vi "QCameraV1_0.vi"() -> (0 "stopped":bool)   [LabVIEW 2012]
uses:
  <vilib>/vision/Image Controls.llb/IMAQ Image.ctl
  SubVI/ProSCI Global.vi
  <userlib>/QI_Transition.llb/QCam Grab Abort.vi
  SubVI/ProSCI DebugGlobal.vi
  <userlib>/QCam Color Globals.vi
  <vilib>/vision/NI_Vision_Development_Module.lvlib
panel:
  out "Images Collected":u64
  in  "Blue Gain":u32=1 min=1 step=1
  in  "Red Gain":u32=1 min=1 step=1
  in  "Green Gain":u32=1 min=1 step=1
  in  "Blue Exposure":dbl=483.0
  in  "Red Exposure":dbl=235.0
  in  "Green Exposure":dbl=300.0
  out "Ratio BlueGreen FL":dbl
  out "Ratio RedGreen FL":dbl
  in  "Link Exposures (FL)":bool
  in  "ForwardDelay":dbl=0.04 min=0.04 max=1074000.0 step=0.001 format="%#.3f"
  in  "FLLampOffDelay":dbl=0.04 min=0.04 max=1074000.0 step=0.001 format="%#.3f"
  in  "FLLampOnDelay":dbl=0.04 min=0.04 max=1074000.0 step=0.001 format="%#.3f"
  in  "BFLampOffDelay":dbl=0.04 min=0.04 max=1074000.0 step=0.001 format="%#.3f"
  in  "BFLampOnDelay":dbl=0.04 min=0.04 max=1074000.0 step=0.001 format="%#.3f"
  in  "PreImagingDelay":dbl=0.04 min=0.04 max=1074000.0 step=0.001 format="%#.3f"
  out "FLExposureTime":dbl[](array[numeric]) caption="Set FL Exposure Time (ms)"
  out "CurrentExposureTime":dbl[](array[numeric]) caption="Current Camera\nExposure Time (ms)"
  in  "SetFLExposureTime":bool
  in  "SetBFExpsureTime":bool
  in  "FLExcite6":bool
  out "FLExciteLED6":bool
  in  "FLExcite5":bool
  out "FLExciteLED5":bool
  in  "FLExcite4":bool
  out "FLExciteLED4":bool
  in  "FLExcite3":bool
  out "FLExciteLED3":bool
  in  "FLExcite2":bool
  out "FLExciteLED2":bool
  in  "FLExcite1":bool
  out "FLExciteLED1":bool
  in  "FL Blue Exp":dbl=0.03999999910593033 min=0.03999999910593033 max=1074000.0 step=0.001 format="%#_3f"
  in  "FL Red Exp":dbl=0.04 min=0.04 max=1074000.0 step=0.001 format="%#.3f"
  in  "FL Exp":dbl=0.04 min=0.04 max=1074000.0 step=0.001 format="%#.3f"
  in  "Case Constant\n(See Context Help) 2":bool
  in  "Case Constant\n(See Context Help)":bool=TRUE
  out "Camera Trigger Mode":T1(ring)
  in  "qImage Type":enum32{"Color", "Grayscale"}(radio)
  out "Ratio BlueGreen":dbl
  out "Ratio RedGreen":dbl
  in  "Tab Control":T2(tab)
  in  "Show Real-Time Image":bool
  out "Real-Time Image":T3(plugin-control)
  in  "Last Or Last Last":enum32{"Last", "Last Last"}(radio)
  in  "Last Display Type":enum32{"Color", "Grayscale"}(radio)
  out "Last Image":T3(plugin-control)
  out "Stream":bool
  out "StatusgGrabImage":bool
  out "Last Last Color":T3
  out "Last Last Mono":T3
  out "Last ColorImage":T3
  out "Last MonoImage":T3
  out "ColorImage":T3
  out "MonoImage":T3
  in  "Snap":bool
  out "TypeChanged":bool
  out "FirstPass":bool
  out "qSerial No":string
  out "last image":errorcluster
  in  "Link Exposures (BF)":bool
  in  "User Blue Exp":dbl=0.03999999910593033 min=0.03999999910593033 max=1074000.0 step=0.001 format="%#_3f"
  in  "User Red Exp":dbl=0.04 min=0.04 max=1074000.0 step=0.001 format="%#.3f"
  in  "White Balance":bool
  in  "Auto Expose":bool
  in  "User Exp":dbl=0.04 min=0.04 max=1074000.0 step=0.001 format="%#.3f"
  in  "Stop Button":bool
  # "CAMERA DISPLAY"
  # "Fluorescence Excitation Filters"
  # "Choice"
  # "Active"
  # "Filter 1"
  # "Filter 2"
  # "Filter 3"
  # "Filter 4"
  # "Filter 5"
  # "Filter 6"
  # "Waiting Scheme (Addition to Exp Time)"
  # "Forward Delay"
  # "msec"
  # "Delay before\nImaging"
  # "msec"
  # "BF Lamp on Delay"
  # "msec"
  # "BF  Lamp off Delay"
  # "msec"
  # "FL  Lamp on Delay"
  # "msec"
  # "FL  Lamp off Delay"
  # "msec"
  # "msec"
  # "msec"
  # "BF Exposure"
  # "FL Exposure"
  # "BF Exposure (Red)"
  # "FL Exposure (Red)"
  # "msec"
  # "msec"
  # "msec"
  # "BF Exposure (Blue)"
  # "FL Exposure (Blue)"
  # "msec"
  # "Display"
  # "Image"
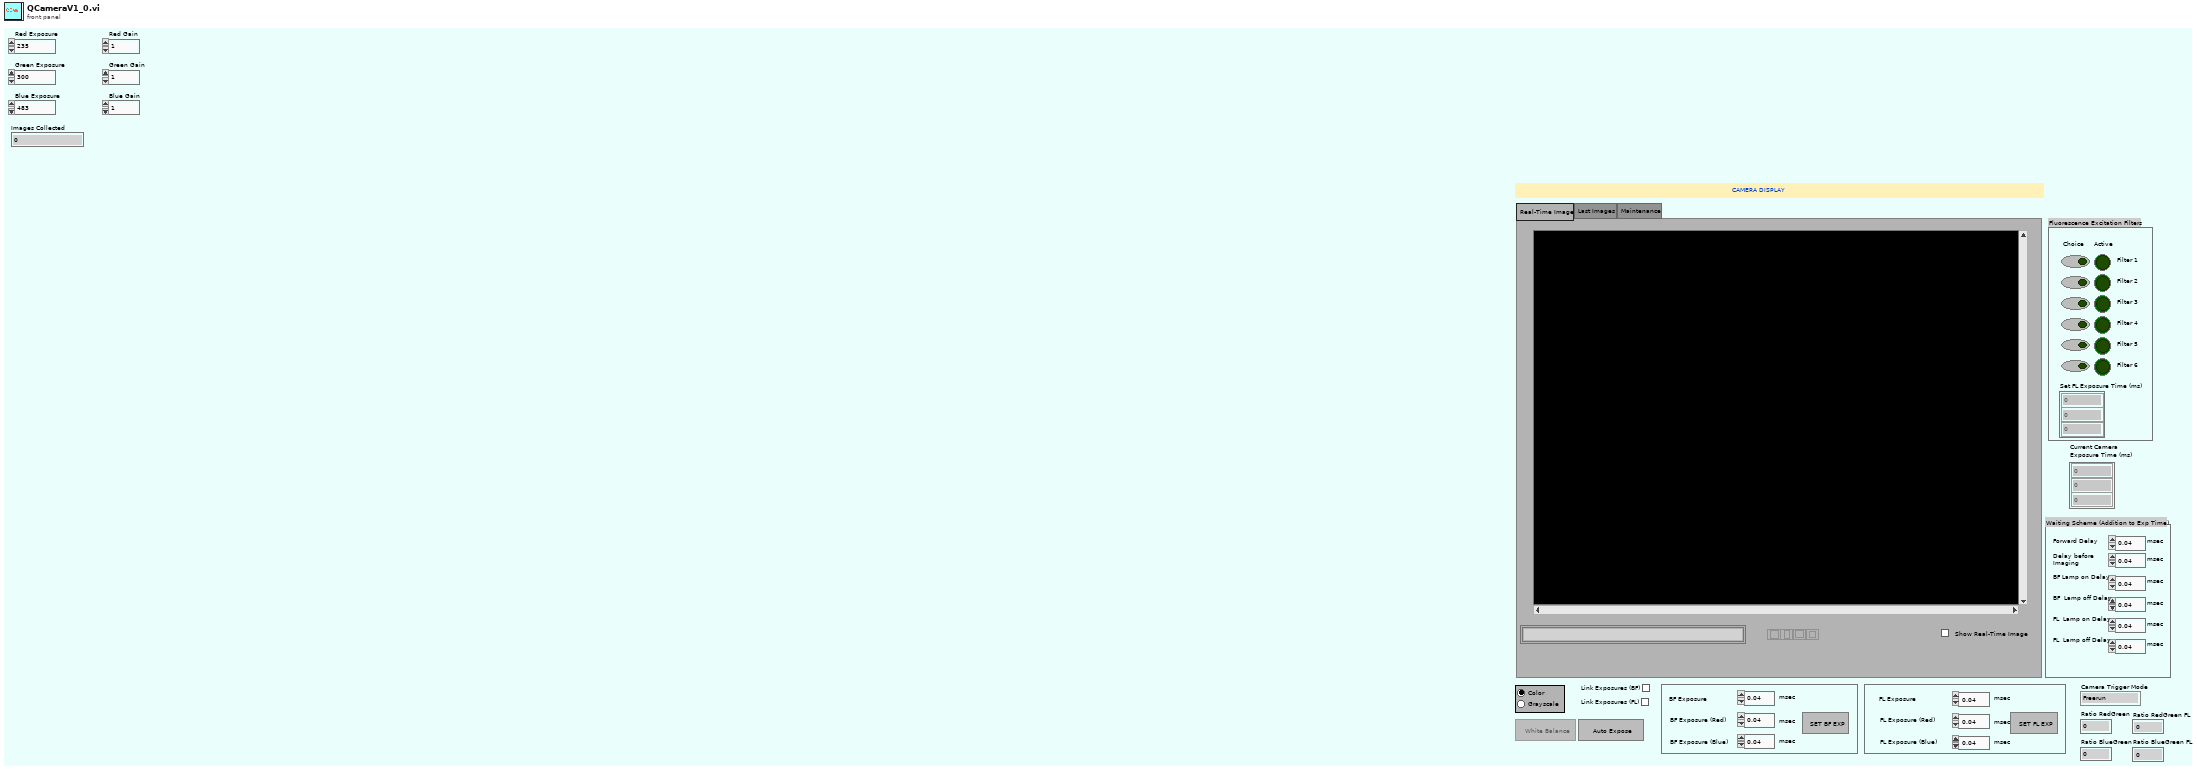
[diagram p1: front panel]
types:
  T1 = enum32{"Freerun", "Edge hi", "Edge low", "Pulse hi", "Pulse low", "Software"}
  T2 = enum32{"Real-Time Image", "Last Images", "Maintenance"}
  T3 = typedef "IMAQ Image.ctl" = refnum<image>
  T4 = typedef "LVRectTypeDef.ctl" = cluster{"Left":i16, "Top":i16, "Right":i16, "Bottom":i16}
  T5 = typedef "Image Type" = u32
  T6 = cluster{"Global Rectangle":i32[], "Contours":cluster{"Contour Type":u32, "ROI Type":u32, "Points":i32[]}[]}
  T7 = cluster{"Green Gain":u32, "Red Gain":u32, "Blue Gain":u32}
  T8 = cluster{"Green Exposure":dbl, "Red Exposure":dbl, "Blue Exposure":dbl}
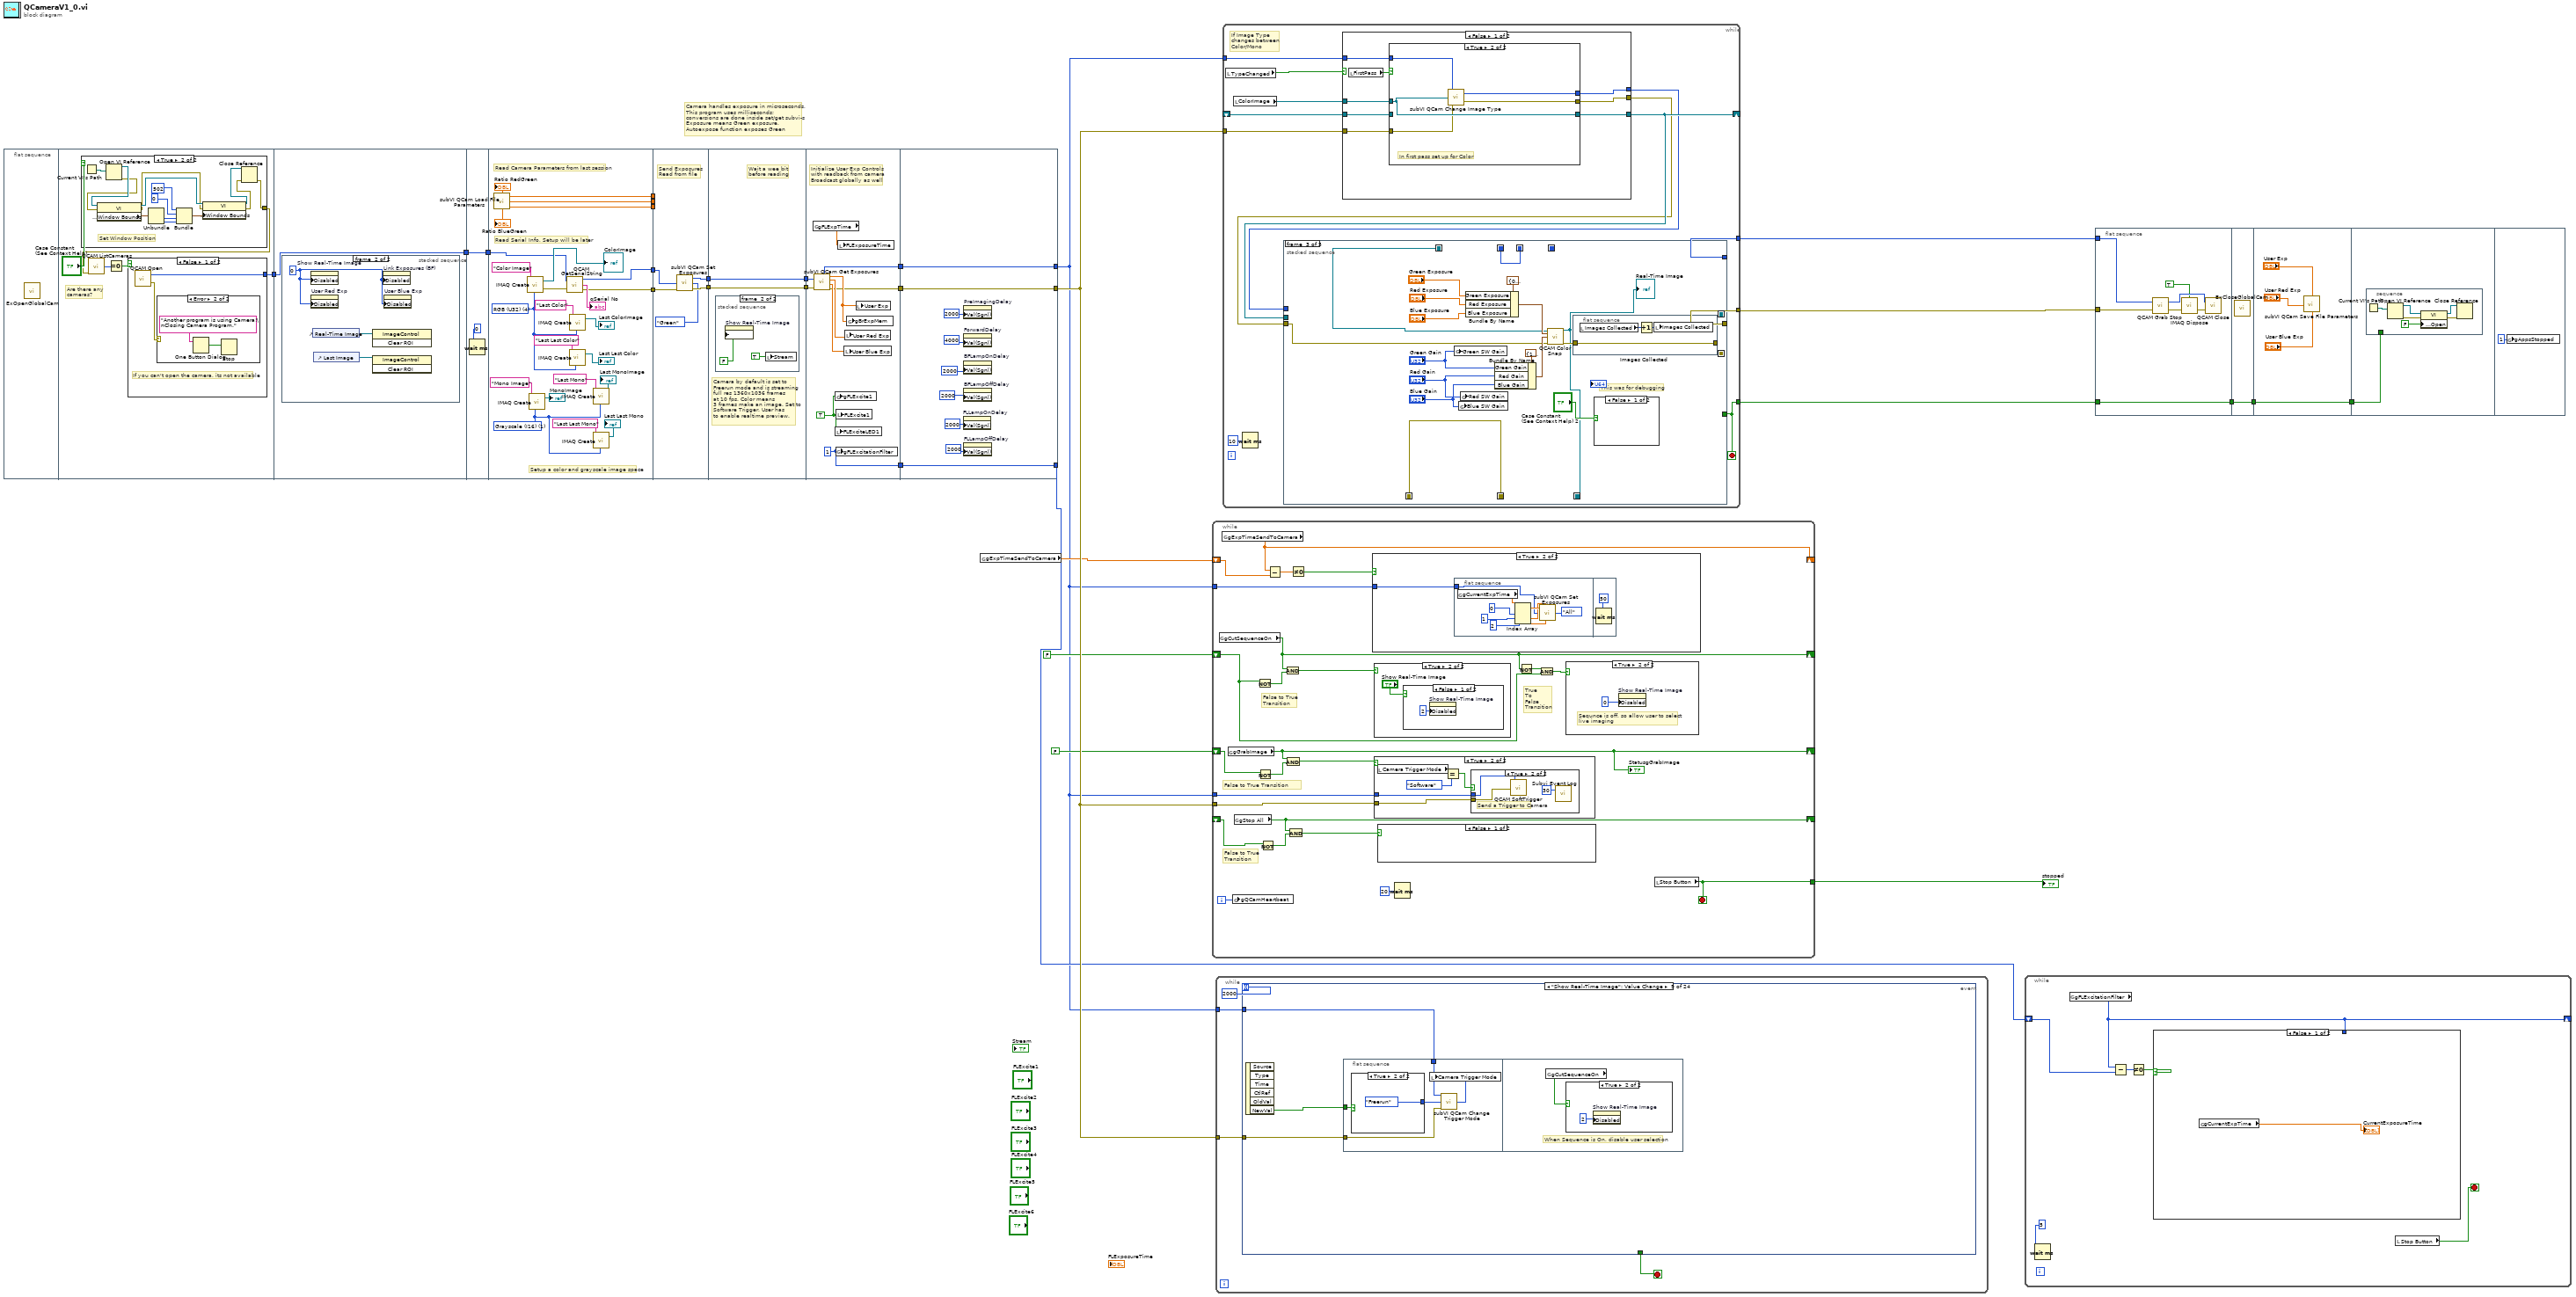
[diagram p0: block diagram]
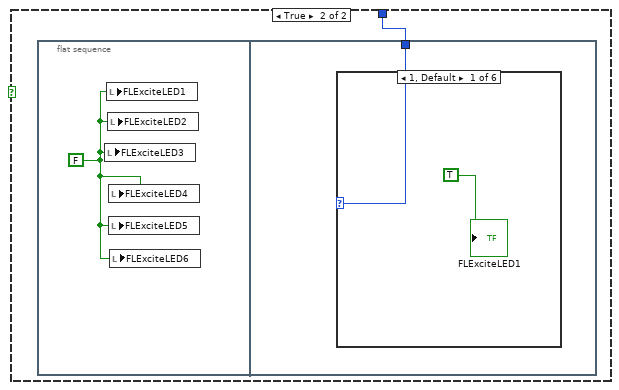
[diagram p2: hidden frame]
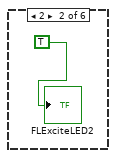
[diagram p3: hidden frame]
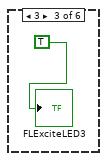
[diagram p4: hidden frame]
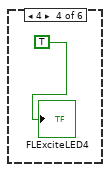
[diagram p5: hidden frame]
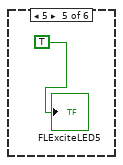
[diagram p6: hidden frame]
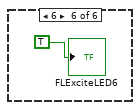
[diagram p7: hidden frame]
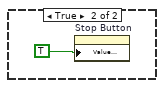
[diagram p8: hidden frame]
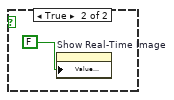
[diagram p13: hidden frame]
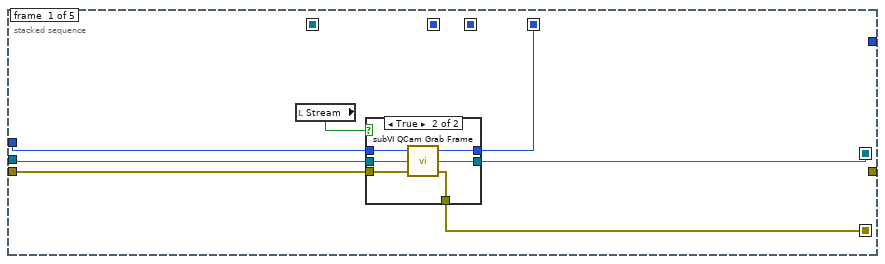
[diagram p15: hidden frame]
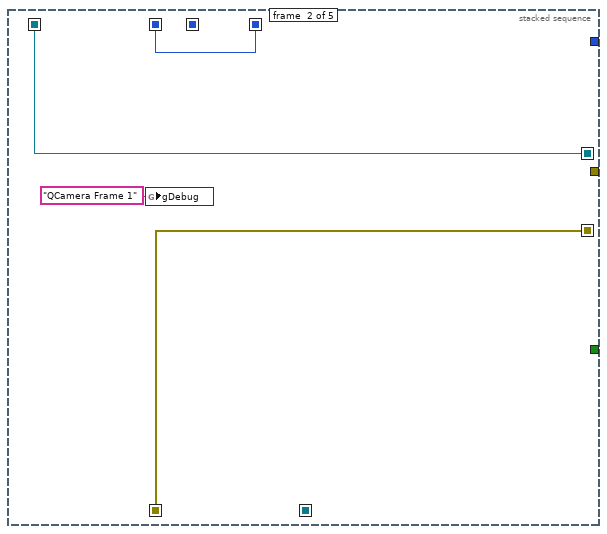
[diagram p17: hidden frame]
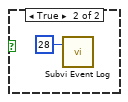
[diagram p18: hidden frame]
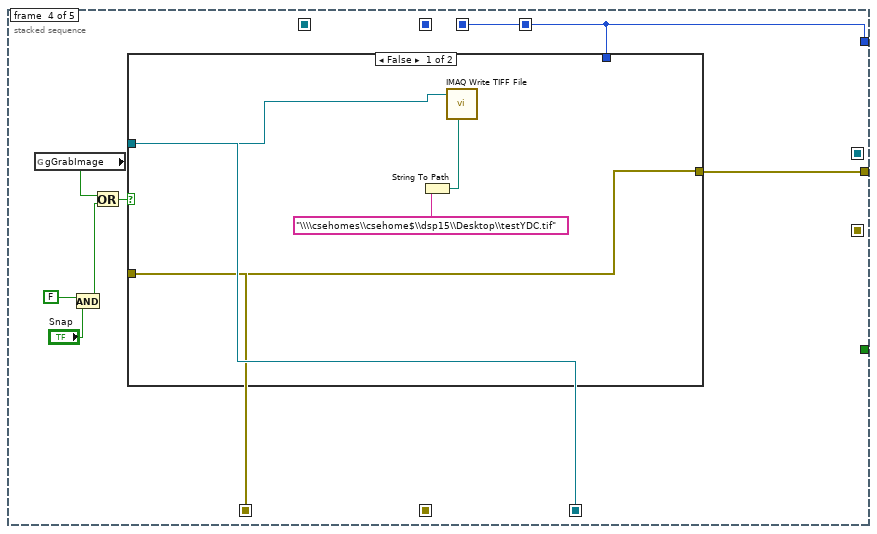
[diagram p19: hidden frame]
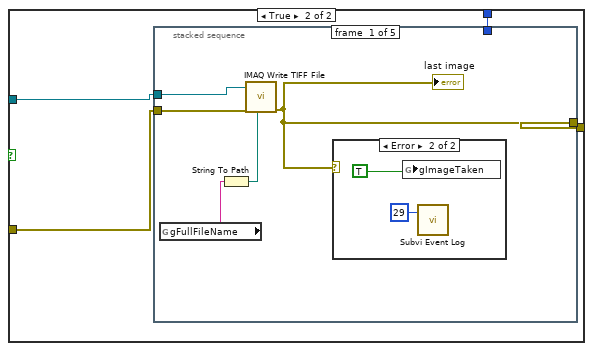
[diagram p20: hidden frame]
diagram:
  # "Camera handles exposure in microseconds,\nThis program uses milliseconds;\nconversions are done inside set/get subvi-s\nExposure means Green exposure,\nAutoexpose function exposes Green"
  n1 = flat-sequence {
    tunnel: [w31] -> w11
    tunnel: [w54] -> w12
    tunnel: w11 -> [w54]
    tunnel: [w61] -> w13
    tunnel: w12 -> [w61]
    tunnel: [w72] -> w28
    tunnel: [w70] -> w27
    tunnel: [w80] -> w26
    tunnel: [w79] -> w25
    tunnel: [w78] -> w24
    tunnel: w13 -> [w63]
    tunnel: w28 -> [w91]
    tunnel: w27 -> [w90]
    tunnel: w26 -> [_]
    tunnel: w25 -> [_]
    tunnel: w24 -> [_]
    tunnel: [w89] -> w22
    tunnel: [w88] -> w20
    tunnel: [w93] -> w23
    tunnel: w22 -> [w93]
    tunnel: [w92] -> w21
    tunnel: w20 -> [w92]
    tunnel: w23 -> [w106]
    tunnel: w21 -> [w105]
    tunnel: [w101] -> w5
    tunnel: [w100] -> w4
    tunnel: [w98] -> w3
    tunnel: [w113] -> w7
    tunnel: [w114] -> w17
    tunnel: [w115] -> w6
    tunnel: w5 -> [w115]
    tunnel: w4 -> [w114]
    tunnel: w3 -> [w113]
    frame #0 {
      n2 = call "ExOpenGlobalCam.vi"() -> ()  [unwired: 1 in]
    }
    frame #1 {
      # "Are there any\ncameras?"
      n3 = case shown="True" "Case Constant\n(See Context Help)" {
        tunnel: [_ w40] -> w29
        frame False {
        }
        frame True {
          # "Set Window Position"
          n4 = Current VI's Path() -> (path=w47:path)
          n5 = Open VI Reference(vi path=w47) -> (vi reference=w46:refnum<vi>, error out=w45:errorcluster)  [unwired: 1 in, 4 out]
          n6 = property class="VI"(reference=w46, error in=w45) -> (reference out=w44:refnum<vi>, error out=w43:errorcluster, "Front Panel Window:Window Bounds"=w53:T4)
          n7 = Unbundle(w53) -> ("Right"=w50:i16, "Bottom"=w51:i16)  [unwired: 2 out]
          n8 = Bundle(i16 502, i16 0, "Right"=w50, "Bottom"=w51) -> (w52:cluster{i16, i16, "Right":i16, "Bottom":i16})  [unwired: 1 out]
          n9 = property class="VI"(reference=w44, error in=w43, "Front Panel Window:Window Bounds"=w52) -> (reference out=w42:refnum<vi>, error out=w41:errorcluster)
          n10 = Close Reference(reference=w42, error in (no error)=w41) -> (error out=w40:errorcluster)
        }
      }
      n11 = call "QCAM ListCameras.vi"("error in (no error)"=w29) -> ("Number of cameras"=w30:u32)  [unwired: 2 out]
      n12 = Equal To 0?(x=w30) -> (x = 0?=w32:bool)
      n13 = case shown="False" w32 {
        tunnel: [w34 _] -> w31
        frame False {
          # "If you can't open the camera, its not available"
          n14 = call <userlib>:"QCAM Open.vi"() -> ("error out"=w35:errorcluster, "cameraId out"=w34:u32)  [unwired: 2 in]
          n15 = case shown="Error" w35 {
            frame No Error {
            }
            frame Error {
              n16 = One Button Dialog(message="Another program is using Camera!\nClosing Camera Program.") -> (true=w36:bool)  [unwired: 1 out]
              n17 = Stop(stop? (T)=w36) -> ()
            }
          }
        }
        frame True {
          n18 = One Button Dialog(message="No Camera Found!\nClosing Camera Program.") -> (true=w38:bool)  [unwired: 1 out]
          n19 = Stop(stop? (T)=w38) -> ()
        }
      }
    }
    frame #2 {
      n20 = stacked-sequence {
        frame #0 {
          w56 = 0
          w55 = FALSE
          n21 = local write "qImage Type"(w56) -> ()
          n22 = global write "ProSCI Global.vi" "gImageMono"(w55) -> ()
          n23 = local write "Link Exposures (BF)"(w55) -> ()
          n24 = local write "Stop Button"(w55) -> ()
          n25 = local write "stopped"(w55) -> ()
          "FirstPass" <- TRUE
          "Camera Trigger Mode" <- w56
        }
        frame #1 {
          w60 = 0
          n26 = property on="Show Real-Time Image" class="Bool (strict)"("Disabled"=w60) -> ()  [unwired: 2 in, 2 out]
          n27 = property on="User Red Exp" class="DigNum (strict)"("Disabled"=w60) -> ()  [unwired: 2 in, 2 out]
          n28 = control-ref of="Real-Time Image"() -> (w59:refnum<vi>)
          n29 = control-ref of="Last Image"() -> (w58:refnum<vi>)
          n30 = invoke class="ImageControl" method="Clear ROI"(reference=w59) -> ()  [unwired: 2 in, 3 out]
          n31 = invoke class="ImageControl" method="Clear ROI"(reference=w58) -> ()  [unwired: 2 in, 3 out]
          n32 = property on="Link Exposures (BF)" class="Bool (strict)"("Disabled"=w60) -> ()  [unwired: 2 in, 2 out]
          n33 = property on="User Blue Exp" class="DigNum (strict)"("Disabled"=w60) -> ()  [unwired: 2 in, 2 out]
        }
      }
    }
    frame #3 {
      n34 = Wait (ms)(milliseconds to wait=0) -> ()  [unwired: 1 out]
    }
    frame #4 {
      w66 = T5 1 items=["Grayscale (U8)", "Grayscale (I16)", "Grayscale (SGL)", "Complex (CSG)", "RGB (U32)", "HSL (U32)", "RGB (U64)"] ("Image Type")
      w68 = T5 4 items=["Grayscale (U8)", "Grayscale (I16)", "Grayscale (SGL)", "Complex (CSG)", "RGB (U32)", "HSL (U32)", "RGB (U64)"] ("Image Type")
      # "Setup a color and grayscale image space"
      # "Read Serial Info, Setup will be later"
      # "Read Camera Parameters from last session"
      n35 = call "subVI QCam Load File Parameters.vi"() -> ("Ratio RedGreen"=→"Ratio RedGreen":dbl, "Ratio BlueGreen"=→"Ratio BlueGreen":dbl, "exposure"=w80:dbl, "exposure Red"=w79:dbl, "exposure Blue"=w78:dbl)
      n36 = call "IMAQ Create"("Image Name"="Color Image", "Image Type"=w68) -> ("New Image"=→"ColorImage":T3, "error out"=w73:errorcluster)  [unwired: 2 in, 1 out]
      n37 = call "IMAQ Create"("Image Name"="Mono Image", "Image Type"=w66) -> ("New Image"=→"MonoImage":T3)  [unwired: 2 in, 2 out]
      n38 = call "QCAM GetSerialString.vi"("cameraId"=w63, "error in (no error)"=w73) -> ("cameraId out"=w72:u32, "value out"=→"qSerial No":string, "error out"=w70:errorcluster)
      n39 = call "IMAQ Create"("Image Name"="Last Last Color", "Image Type"=w68) -> ("New Image"=→"Last Last Color":T3)  [unwired: 2 in, 2 out]
      n40 = call "IMAQ Create"("Image Name"="Last Color", "Image Type"=w68) -> ("New Image"=→"Last ColorImage":T3)  [unwired: 2 in, 2 out]
      n41 = call "IMAQ Create"("Image Name"="Last Mono", "Image Type"=w66) -> ("New Image"=→"Last MonoImage":T3)  [unwired: 2 in, 2 out]
      n42 = call "IMAQ Create"("Image Name"="Last Last Mono", "Image Type"=w66) -> ("New Image"=→"Last Last Mono":T3)  [unwired: 2 in, 2 out]
    }
    frame #5 {
      # "Send Exposures\nRead from file"
      n43 = call "subVI QCam Set Exposures.vi"("cameraId In"=w91, "error In"=w90, "Set Which Exposure"=enum16{"All", "Green", "Red", "Blue"}."Green") -> ("cameraId out"=w89:u32, "error out"=w88:errorcluster)  [unwired: 3 in]
    }
    frame #6 {
      # "Camera by default is set to\nFreerun mode and is streaming\nfull res 1360x1036 frames\nat 10 fps. Color means\n3 frames make an image. Set to\nSoftware Trigger. User has\nto enable realtime preview."
      # "Wait a wee bit\nbefore reading"
      n44 = stacked-sequence {
        frame #0 {
          n45 = Wait (ms)(milliseconds to wait=100) -> ()  [unwired: 1 out]
        }
        frame #1 {
          n46 = property on="Show Real-Time Image" class="Bool (strict)"("Value (Signaling)"=FALSE) -> ()  [unwired: 2 in, 2 out]
          n47 = local write "Stream"(TRUE ("Stream")) -> ()
        }
      }
    }
    frame #7 {
      w99 = TRUE
      w98 = 1
      # "Initialize User Exp Controls\nwith readback from camera\nBroadcast globally as well"
      n48 = global read "ProSCI Global.vi" "gFLExpTime"() -> (w97:dbl[])
      n49 = call "subVI QCam Get Exposures.vi"("error In"=w105, "cameraId In"=w106) -> ("error out"=w100:errorcluster, "qExposure Blue"=w104:dbl, "qExposure Red"=w103:dbl, "qExposure"=w102:dbl, "cameraId out"=w101:u32)
      n50 = global write "ProSCI Global.vi" "gFLExcite1"(w99) -> ()
      n51 = local write "FLExciteLED1"(w99) -> ()
      n52 = global write "ProSCI Global.vi" "gFLExcitationFilter"(w98) -> ()
      n53 = local write "FLExcite1"(w99) -> ()
      n54 = local write "FLExposureTime"(w97) -> ()
      n55 = local write "User Blue Exp"(w104) -> ()
      n56 = local write "User Red Exp"(w103) -> ()
      n57 = global write "ProSCI Global.vi" "gBrExpMem"(w102) -> ()
      n58 = local write "User Exp"(w102) -> ()
    }
    frame #8 {
      n59 = property on="FLLampOnDelay" class="DigNum (strict)"("Val(Sgnl)"=2000) -> ()  [unwired: 2 in, 2 out]
      n60 = property on="PreImagingDelay" class="DigNum (strict)"("Val(Sgnl)"=2000) -> ()  [unwired: 2 in, 2 out]
      n61 = property on="ForwardDelay" class="DigNum (strict)"("Val(Sgnl)"=4000) -> ()  [unwired: 2 in, 2 out]
      n62 = property on="BFLampOnDelay" class="DigNum (strict)"("Val(Sgnl)"=2000) -> ()  [unwired: 2 in, 2 out]
      n63 = property on="BFLampOffDelay" class="DigNum (strict)"("Val(Sgnl)"=2000) -> ()  [unwired: 2 in, 2 out]
      n64 = property on="FLLampOffDelay" class="DigNum (strict)"("Val(Sgnl)"=2000) -> ()  [unwired: 2 in, 2 out]
    }
  }
  n65 = global read "ProSCI Global.vi" "gExpTimeSendToCamera"() -> (w8:dbl)
  n66 = while {
    shift-right: [w117] -> _
    shift-left: w8 -> [w138]
    shift-right: [w133] -> _
    shift-left: FALSE -> [w131]
    shift-right: [w118] -> _
    shift-left: FALSE -> [w129]
    tunnel: w6 -> [w127]
    tunnel: w17 -> [w126]
    tunnel: [w124] -> w14
    shift-right: [w122] -> _
    shift-left: _ -> [w121]
    tunnel: w6 -> [w116]
    i -> [w125]
    stop <- w124 stop-if-true
    # "False to True\nTransition"
    # "False to True Transition"
    # "True\nTo\nFalse\nTransition"
    # "False to True\nTransition"
    n67 = global read "ProSCI Global.vi" "gCutSequenceOn"() -> (w133:bool)
    n68 = global read "ProSCI Global.vi" "gExpTimeSendToCamera"() -> (w117:dbl)
    n69 = global read "ProSCI Global.vi" "gGrabImage"() -> (w118:bool)
    "StatusgGrabImage" <- w118
    n70 = global write "ProSCI Global.vi" "gQCamHeartbeat"(w125) -> ()
    n71 = global read "ProSCI Global.vi" "gStop All"() -> (w122:bool)
    n72 = Not(x=w131) -> (.not. x?=w136:bool)
    n73 = Not(x=w129) -> (.not. x?=w130:bool)
    n74 = Not(x=w121) -> (.not. x?=w123:bool)
    n75 = Subtract(x=w117, y=w138) -> (x-y=w139:dbl)
    n76 = And(x=w133, y=w136) -> (x .and. y?=w135:bool)
    n77 = And(x=w118, y=w130) -> (x .and. y?=w128:bool)
    n78 = And(x=w122, y=w123) -> (x .and. y?=w120:bool)
    n79 = Not Equal To 0?(x=w139) -> (x != 0?=w137:bool)
    n80 = case shown="True" w137 {
      tunnel: w116 -> [_ w153]
      frame False {
      }
      frame True {
        n81 = flat-sequence {
          tunnel: w153 -> [w154]
          frame #0 {
            n82 = global read "ProSCI Global.vi" "gCurrentExpTime"() -> (w162:dbl[])
            n83 = Index Array(array=w162, index #1=0, index #2=1, index #3=2) -> (element #1=w157:dbl, element #2=w156:dbl, element #3=w155:dbl)
            n84 = call "subVI QCam Set Exposures.vi"("qExposure"=w157, "qExposure Red"=w156, "cameraId In"=w154, "qExposure Blue"=w155, "Set Which Exposure"=enum16{"All", "Green", "Red", "Blue"}."All") -> ()  [unwired: 1 in, 2 out]
          }
          frame #1 {
            n85 = Wait (ms)(milliseconds to wait=u32 50) -> ()  [unwired: 1 out]
          }
        }
      }
    }
    n86 = case shown="True" w135 {
      frame False {
      }
      frame True {
        n87 = case shown="False" "Show Real-Time Image" {
          frame False {
            n88 = property on="Show Real-Time Image" class="Bool (strict)"("Disabled"=u8 2) -> ()  [unwired: 2 in, 2 out]
          }
          frame True {
            n89 = property on="Show Real-Time Image" class="Bool (strict)"("Value (Signaling)"=FALSE) -> ()  [unwired: 2 in, 2 out]
          }
        }
      }
    }
    n90 = case shown="True" w128 {
      tunnel: w127 -> [_ w145]
      tunnel: w126 -> [_ w144]
      frame False {
      }
      frame True {
        n91 = local read "Camera Trigger Mode"() -> (w143:T1)
        n92 = Equal?(x=w143, y=T1."Software" ("Trigger Mode")) -> (x = y?=w141:bool)
        n93 = case shown="True" w141 {
          tunnel: w145 -> [_ w148]
          tunnel: w144 -> [_ w147]
          frame False {
          }
          frame True {
            # "Send a Trigger to Camera"
            n94 = call "QCAM SoftTrigger.vi"("error in (no error)"=w147, "cameraId"=w148) -> ()  [unwired: 2 out]
            n95 = call "Subvi Event Log.vi"("EventNum"=u32 30) -> ()  [unwired: 1 in]
          }
        }
      }
    }
    n96 = case shown="False" w120 {
      frame False {
      }
      frame True {
        n97 = property on="Stop Button" class="Bool (strict)"("Value (Signaling)"=TRUE) -> ()  [unwired: 2 in, 2 out]
      }
    }
    n98 = Wait (ms)(milliseconds to wait=u32 20) -> ()  [unwired: 1 out]
    n99 = Not(x=w133) -> (.not. x?=w132:bool)
    n100 = And(x=w132, y=w131) -> (x .and. y?=w134:bool)
    n101 = case shown="True" w134 {
      frame False {
      }
      frame True {
        # "Sequnce is off, so allow user to select\nlive imaging"
        n102 = property on="Show Real-Time Image" class="Bool (strict)"("Disabled"=0) -> ()  [unwired: 2 in, 2 out]
      }
    }
    n103 = local read "Stop Button"() -> (w124:bool)
  }
  "stopped" <- w14
  n104 = while {
    tunnel: w6 -> [w166]
    tunnel: w17 -> [w165]
    stop <- w164 stop-if-true
    n105 = event shown="[8] \"Show Real-Time Image\": Value Change" {
      selector: _ -> [_ _ _ _ _ _ _ _ _ _ _ _ _ _ _ _ _ _ _ _ _ _ _ _]
      dyn-events: _ -> [_ _ _ _ _ _ _ _ _ _ _ _ _ _ _ _ _ _ _ _ _ _ _ _]
      timeout: 2000 -> [_ _ _ _ _ _ _ _ _ _ _ _ _ _ _ _ _ _ _ _ _ _ _ _]
      tunnel: w166 -> [_ w168 w193 _ _ _ _ _ w274 w286 _ _ _ _ _ _ w333 w396 _ _ _ _ _ _]
      tunnel: w165 -> [_ _ w192 _ _ _ _ _ w273 w285 _ _ _ _ _ _ w332 w395 _ _ _ _ _ _]
      tunnel: [_ _ _ _ _ w248 _ _ _ _ _ _ _ _ _ _ _ _ _ _ _ _ _ _] -> w164
      event Timeout {
        n106 = event-data() -> ()  [unwired: 3 out]
      }
      event "Auto Expose": Mouse Down {
        n107 = event-data() -> ()  [unwired: 3 out]
        n108 = stacked-sequence {
          seq-local: [w171 _ _ _] -> [_ _ w189 _]
          seq-local: [_ _ w188 _] -> [_ _ _ _]
          tunnel: w168 -> [w170 _ w190 _]
          frame #0 {
            # "Call Autoexpose function"
            n109 = flat-sequence {
              tunnel: w170 -> [w173]
              tunnel: [w173] -> w169
              tunnel: [w175] -> w171
              tunnel: w169 -> [w174]
              frame #0 {
                n110 = local write "Stream"(FALSE ("Stream")) -> ()
              }
              frame #1 {
                n111 = property on="Real-Time Image" class="ImageControl"() -> ("ROI"=w183:T6)  [unwired: 2 in, 2 out]
                n112 = Unbundle(w183) -> ("Global Rectangle"=w182:i32[])  [unwired: 1 out]
                n113 = Index Array(array=w182) -> (element #1=w180:i32, element #2=w178:i32, element #4=w181:i32, element #5=w177:i32)  [unwired: 5 in, 1 out]
                n114 = Subtract(x=w181, y=w180) -> (x-y=w179:i32)
                n115 = Subtract(x=w177, y=w178) -> (x-y=w176:i32)
                n116 = call "QCAM AutoExpose.vi"("xOrig"=w180, "cameraId"=w174, "yOrig"=w178, "Width"=w179, "height"=w176) -> ("error out"=w175:errorcluster)  [unwired: 1 in, 2 out]
              }
            }
          }
          frame #1 {
            n117 = Wait (ms)(milliseconds to wait=u32 50) -> ()  [unwired: 1 out]
          }
          frame #2 {
            # "Read back the green exposure (AE only works on Green)"
            n118 = call "subVI QCam Get Exposures.vi"("error In"=w189, "cameraId In"=w190) -> ("qExposure Blue"=w186:dbl, "qExposure Red"=w187:dbl, "qExposure"=w188:dbl)  [unwired: 2 out]
            n119 = Build Array(w188, w187, w186) -> (w185:dbl[])
            n120 = global write "ProSCI Global.vi" "gCurrentExpTime"(w185) -> ()
          }
          frame #3 {
            n121 = local write "Stream"(TRUE ("Stream")) -> ()
          }
        }
      }
      event "White Balance": Mouse Down {
        n122 = event-data() -> ()  [unwired: 3 out]
        n123 = stacked-sequence {
          tunnel: w193 -> [w207 _]
          tunnel: w192 -> [w206 _]
          frame #0 {
            n124 = property on="Real-Time Image" class="ImageControl"() -> ("ROI"=w205:T6)  [unwired: 2 in, 2 out]
            n125 = Unbundle(w205) -> ("Global Rectangle"=w204:i32[])  [unwired: 1 out]
            n126 = Index Array(array=w204) -> (element #1=w200:i32, element #2=w199:i32, element #3=w195:i32, element #4=w194:i32)  [unwired: 4 in]
            n127 = Subtract(x=w195, y=w200) -> (x-y=w198:i32)
            n128 = Equal To 0?(x=w198) -> (x = 0?=w202:bool)
            n129 = local write "Stream"(FALSE ("Stream")) -> ()
            n130 = Subtract(x=w194, y=w199) -> (x-y=w197:i32)
            n131 = Equal To 0?(x=w197) -> (x = 0?=w203:bool)
            n132 = Or(x=w203, y=w202) -> (x .or. y?=w201:bool)
            n133 = case shown="False" w201 {
              tunnel: w207 -> [w213 _]
              tunnel: w206 -> [w212 _]
              tunnel: w200 -> [w211 _]
              tunnel: w199 -> [w210 _]
              tunnel: w198 -> [w209 _]
              tunnel: w197 -> [w208 _]
              frame False {
                n134 = stacked-sequence {
                  tunnel: w213 -> [w219 w227]
                  tunnel: w212 -> [w218 w228]
                  tunnel: w211 -> [w217 _]
                  tunnel: w210 -> [w216 _]
                  tunnel: w209 -> [w215 _]
                  tunnel: w208 -> [w214 _]
                  frame #0 {
                    # "Do a white balance on the region of interest defined on\nReal Time image"
                    n135 = call "QCAM WhiteBalance.vi"("xOrig"=w217, "cameraId"=w219, "yOrig"=w216, "width"=w215, "error in (no error)"=w218, "height"=w214) -> ()  [unwired: 3 out]
                  }
                  frame #1 {
                    # "Update ratios for color if linked is True"
                    n136 = local read "qImage Type"() -> (w223:enum32{"Color", "Grayscale"})
                    n137 = local read "Link Exposures (BF)"() -> (w222:bool)
                    n138 = call "subVI QCam Get Exposures.vi"("error In"=w228, "cameraId In"=w227) -> ("qExposure Blue"=w224:dbl, "qExposure Red"=w225:dbl, "qExposure"=w226:dbl)  [unwired: 2 out]
                    n139 = local write "User Blue Exp"(w224) -> ()
                    n140 = local write "User Exp"(w226) -> ()
                    n141 = local write "User Red Exp"(w225) -> ()
                    n142 = Equal To 0?(x=w223) -> (x = 0?=w221:bool)
                    n143 = And(x=w222, y=w221) -> (x .and. y?=w220:bool)
                    n144 = case shown="True" w220 {
                      tunnel: w226 -> [_ w233]
                      tunnel: w225 -> [_ w232]
                      tunnel: w224 -> [_ w231]
                      frame False {
                      }
                      frame True {
                        n145 = call "subVI QCam Calculate Exposure Ratios.vi"("exposure Blue"=w231, "exposure Red"=w232, "exposure"=w233) -> ("Ratio BlueGreen"=w229:dbl, "Ratio RedGreen"=w230:dbl)
                        n146 = local write "Ratio BlueGreen"(w229) -> ()
                        n147 = local write "Ratio RedGreen"(w230) -> ()
                      }
                    }
                  }
                }
              }
              frame True {
                n148 = One Button Dialog(message="ROI Not Selected.\nWhite Balance Not Possible.") -> ()  [unwired: 2 out]
              }
            }
          }
          frame #1 {
            n149 = local write "Stream"(TRUE ("Stream")) -> ()
          }
        }
      }
      event "Link Exposures (BF)": Value Change {
        n150 = event-data() -> ("NewVal"=w236:bool)  [unwired: 6 out]
        n151 = case shown="True" w236 {
          frame False {
          }
          frame True {
            n152 = local read "User Blue Exp"() -> (w239:dbl)
            n153 = local read "User Red Exp"() -> (w240:dbl)
            n154 = local read "User Exp"() -> (w241:dbl)
            n155 = call "subVI QCam Calculate Exposure Ratios.vi"("exposure Blue"=w239, "exposure Red"=w240, "exposure"=w241) -> ("Ratio BlueGreen"=w237:dbl, "Ratio RedGreen"=w238:dbl)
            n156 = local write "Ratio RedGreen"(w238) -> ()
            n157 = local write "Ratio BlueGreen"(w237) -> ()
          }
        }
      }
      event "Link Exposures (FL)": Value Change {
        n158 = event-data() -> ("NewVal"=w242:bool)  [unwired: 6 out]
        n159 = case shown="True" w242 {
          frame False {
          }
          frame True {
            n160 = local read "FL Exp"() -> (w244:dbl)
            n161 = local read "FL Red Exp"() -> (w245:dbl)
            n162 = local read "FL Blue Exp"() -> (w246:dbl)
            n163 = Divide(x=w245, y=w244) -> (x/y=→"Ratio RedGreen FL":dbl)
            n164 = Divide(x=w246, y=w244) -> (x/y=→"Ratio BlueGreen FL":dbl)
          }
        }
      }
      event "Stop Button": Value Change {
        n165 = event-data() -> ()  [unwired: 7 out]
        n166 = flat-sequence {
          tunnel: ["Stop Button"] -> w248
          frame #0 {
            n167 = global write "QCam Grab Abort.vi" "Grab Abort"(TRUE) -> ()
          }
          frame #1 {
          }
        }
      }
      event "Last Display Type": Value Change {
        n168 = event-data() -> ("NewVal"=w253:enum32{"Color", "Grayscale"})  [unwired: 6 out]
        n169 = local read "Last Or Last Last"() -> (w251:enum32{"Last", "Last Last"})
        n170 = case shown="\"Grayscale\"" w253 {
          tunnel: [w255 w259] -> w252
          tunnel: w251 -> [w254 w258]
          frame "Color", Default {
            n171 = case shown="\"Last Last\"" w254 {
              tunnel: [w256 w257] -> w255
              frame "Last", Default {
                n172 = local read "Last ColorImage"() -> (w256:T3)
              }
              frame "Last Last" {
                n173 = local read "Last Last Color"() -> (w257:T3)
              }
            }
          }
          frame "Grayscale" {
            n174 = case shown="\"Last Last\"" w258 {
              tunnel: [w260 w261] -> w259
              frame "Last", Default {
                n175 = local read "Last MonoImage"() -> (w260:T3)
              }
              frame "Last Last" {
                n176 = local read "Last Last Mono"() -> (w261:T3)
              }
            }
          }
        }
        n177 = local write "Last Image"(w252) -> ()
      }
      event "Last Or Last Last": Value Change {
        n178 = event-data() -> ("NewVal"=w264:enum32{"Last", "Last Last"})  [unwired: 6 out]
        n179 = case shown="\"Last\", Default" w264 {
          tunnel: "Last Display Type" -> [w266 w270]
          tunnel: [w265 w269] -> w262
          frame "Last", Default {
            n180 = case shown="\"Color\", Default" w266 {
              tunnel: [w267 w268] -> w265
              frame "Color", Default {
                n181 = local read "Last ColorImage"() -> (w267:T3)
              }
              frame "Grayscale" {
                n182 = local read "Last MonoImage"() -> (w268:T3)
              }
            }
          }
          frame "Last Last" {
            n183 = case shown="\"Color\", Default" w270 {
              tunnel: [w271 w272] -> w269
              frame "Color", Default {
                n184 = local read "Last Last Color"() -> (w271:T3)
              }
              frame "Grayscale" {
                n185 = local read "Last Last Mono"() -> (w272:T3)
              }
            }
          }
        }
        n186 = local write "Last Image"(w262) -> ()
      }
      event "Show Real-Time Image": Value Change {
        n187 = event-data() -> ("NewVal"=w275:bool)  [unwired: 6 out]
        n188 = flat-sequence {
          tunnel: w275 -> [w280]
          tunnel: w274 -> [w278]
          tunnel: w273 -> [w277]
          frame #0 {
            n189 = case shown="True" w280 {
              tunnel: [T1."Software" ("Trigger Mode") T1."Freerun" ("Trigger Mode")] -> w279
              frame False {
              }
              frame True {
              }
            }
            n190 = call "subVI QCam Change Trigger Mode.vi"("error in"=w277, "trigger mode"=w279, "cameraId In"=w278) -> ("trigger mode fbk"=w276:T1)  [unwired: 2 out]
            n191 = local write "Camera Trigger Mode"(w276) -> ()
          }
          frame #1 {
            # "When Sequence is On, disable user selection"
            n192 = global read "ProSCI Global.vi" "gCutSequenceOn"() -> (w283:bool)
            n193 = case shown="True" w283 {
              frame False {
              }
              frame True {
                n194 = property on="Show Real-Time Image" class="Bool (strict)"("Disabled"=2) -> ()  [unwired: 2 in, 2 out]
              }
            }
          }
        }
      }
      event "qImage Type": Value Change {
        n195 = event-data() -> ("NewVal"=w287:enum32{"Color", "Grayscale"})  [unwired: 6 out]
        n196 = stacked-sequence {
          tunnel: w287 -> [w292 _ _]
          tunnel: w286 -> [w289 _ _]
          tunnel: w285 -> [w288 _ _]
          frame #0 {
            # "If Image Type has been selected to be\ncolor, enable controls"
            n197 = Equal To 0?(x=w292) -> (x = 0?=w291:bool)
            n198 = case shown="True" w291 {
              tunnel: [2 w294] -> w290
              tunnel: w289 -> [_ w296]
              tunnel: w288 -> [_ w295]
              frame False {
                # "Disable and\nGray Out"
              }
              frame True {
                n199 = stacked-sequence {
                  tunnel: w296 -> [w299 _]
                  tunnel: w295 -> [w298 _]
                  tunnel: [_ 0] -> w294
                  frame #0 {
                    n200 = local read "Link Exposures (BF)"() -> (w297:bool)
                    n201 = case shown="True" w297 {
                      tunnel: w299 -> [_ w301]
                      tunnel: w298 -> [_ w300]
                      frame False {
                      }
                      frame True {
                        n202 = stacked-sequence {
                          seq-local: [w302 _] -> [_ w307]
                          tunnel: w301 -> [w306 w309]
                          tunnel: w300 -> [w305 _]
                          frame #0 {
                            n203 = local read "User Red Exp"() -> (w304:dbl)
                            n204 = call "subVI QCam Set Exposures.vi"("qExposure Red"=w304, "cameraId In"=w306, "error In"=w305, "Set Which Exposure"=enum16{"All", "Green", "Red", "Blue"}."Red") -> ("error out"=w302:errorcluster)  [unwired: 2 in, 1 out]
                          }
                          frame #1 {
                            n205 = local read "User Blue Exp"() -> (w308:dbl)
                            n206 = call "subVI QCam Set Exposures.vi"("cameraId In"=w309, "error In"=w307, "qExposure Blue"=w308, "Set Which Exposure"=enum16{"All", "Green", "Red", "Blue"}."Blue") -> ()  [unwired: 2 in, 2 out]
                          }
                        }
                      }
                    }
                  }
                  frame #1 {
                    # "Enable"
                  }
                }
              }
            }
            n207 = property on="User Red Exp" class="DigNum (strict)"("Disabled"=w290) -> ()  [unwired: 2 in, 2 out]
            n208 = property on="User Blue Exp" class="DigNum (strict)"("Disabled"=w290) -> ()  [unwired: 2 in, 2 out]
            n209 = property on="Link Exposures (BF)" class="Bool (strict)"("Disabled"=w290) -> ()  [unwired: 2 in, 2 out]
            n210 = property on="White Balance" class="Bool"("Disabled"=w290) -> ()  [unwired: 2 in, 2 out]
          }
          frame #1 {
            "TypeChanged" <- TRUE
          }
          frame #2 {
            n211 = global write "QCam Grab Abort.vi" "Grab Abort"(TRUE) -> ()
          }
        }
      }
      event "FLExcite1": Value Change {
        n212 = event-data() -> ("NewVal"=w316:bool)  [unwired: 6 out]
        n213 = global write "ProSCI Global.vi" "gFLExcite1"(w316) -> ()
        n214 = global write "ProSCI Global.vi" "gFLExcitationFilter"(1) -> ()
        n215 = global read "ProSCI Global.vi" "gFLExpTime"() -> (w314:dbl[])
        n216 = local write "FLExposureTime"(w314) -> ()
      }
      event "FLExcite2": Value Change {
        n217 = event-data() -> ("NewVal"=w319:bool)  [unwired: 6 out]
        n218 = global write "ProSCI Global.vi" "gFLExcitationFilter"(2) -> ()
        n219 = global write "ProSCI Global.vi" "gFLExcite2"(w319) -> ()
        n220 = global read "ProSCI Global.vi" "gFLExpTime 2"() -> (w317:dbl[])
        n221 = local write "FLExposureTime"(w317) -> ()
      }
      event "FLExcite3": Value Change {
        n222 = event-data() -> ("NewVal"=w322:bool)  [unwired: 6 out]
        n223 = global write "ProSCI Global.vi" "gFLExcitationFilter"(3) -> ()
        n224 = global write "ProSCI Global.vi" "gFLExcite3"(w322) -> ()
        n225 = global read "ProSCI Global.vi" "gFLExpTime 3"() -> (w320:dbl[])
        n226 = local write "FLExposureTime"(w320) -> ()
      }
      event "FLExcite4": Value Change {
        n227 = event-data() -> ("NewVal"=w325:bool)  [unwired: 6 out]
        n228 = global write "ProSCI Global.vi" "gFLExcitationFilter"(4) -> ()
        n229 = global write "ProSCI Global.vi" "gFLExcite4"(w325) -> ()
        n230 = global read "ProSCI Global.vi" "gFLExpTime 4"() -> (w323:dbl[])
        n231 = local write "FLExposureTime"(w323) -> ()
      }
      event "FLExcite5": Value Change {
        n232 = event-data() -> ("NewVal"=w328:bool)  [unwired: 6 out]
        n233 = global write "ProSCI Global.vi" "gFLExcitationFilter"(5) -> ()
        n234 = global write "ProSCI Global.vi" "gFLExcite5"(w328) -> ()
        n235 = global read "ProSCI Global.vi" "gFLExpTime 5"() -> (w326:dbl[])
        n236 = local write "FLExposureTime"(w326) -> ()
      }
      event "FLExcite6": Value Change {
        n237 = event-data() -> ("NewVal"=w331:bool)  [unwired: 6 out]
        n238 = global write "ProSCI Global.vi" "gFLExcitationFilter"(6) -> ()
        n239 = global write "ProSCI Global.vi" "gFLExcite6"(w331) -> ()
        n240 = global read "ProSCI Global.vi" "gFLExpTime 6"() -> (w329:dbl[])
        n241 = local write "FLExposureTime"(w329) -> ()
      }
      event "SetFLExposureTime": Value Change {
        n242 = event-data() -> ()  [unwired: 7 out]
        n243 = stacked-sequence {
          tunnel: w333 -> [w338 w393 _]
          tunnel: w332 -> [w337 w392 _]
          frame #0 {
            n244 = flat-sequence {
              tunnel: [w343] -> w336
              tunnel: [w342] -> w335
              tunnel: [w341] -> w334
              tunnel: [w356] -> w339
              tunnel: w338 -> [w358]
              tunnel: w337 -> [w357]
              tunnel: w336 -> [w356]
              tunnel: w335 -> [w355]
              tunnel: w334 -> [w354]
              tunnel: w339 -> [w387]
              frame #0 {
                n245 = local write "Stream"(FALSE ("Stream")) -> ()
              }
              frame #1 {
                n246 = case shown="True" "Link Exposures (FL)" {
                  tunnel: [w346 w349] -> w343
                  tunnel: "FL Exp" -> [w346 w349]
                  tunnel: ["FL Red Exp" w353] -> w342
                  tunnel: ["FL Blue Exp" w351] -> w341
                  frame False {
                  }
                  frame True {
                    n247 = local read "Ratio BlueGreen FL"() -> (w350:dbl)
                    n248 = local read "Ratio RedGreen FL"() -> (w352:dbl)
                    n249 = Multiply(x=w349, y=w352) -> (x*y=w353:dbl)
                    n250 = Multiply(x=w349, y=w350) -> (x*y=w351:dbl)
                  }
                }
              }
              frame #2 {
                n251 = global read "ProSCI Global.vi" "gFLExcitationFilter"() -> (w360:i8)
                n252 = call "subVI QCam Set Exposures.vi"("qExposure"=w356, "qExposure Red"=w355, "cameraId In"=w358, "error In"=w357, "qExposure Blue"=w354, "Set Which Exposure"=enum16{"All", "Green", "Red", "Blue"}."All") -> ()  [unwired: 2 out]
                n253 = case shown="6" w360 {
                  tunnel: w356 -> [_ w365 w369 w373 w377 w381 w385]
                  tunnel: w355 -> [_ w364 w368 w372 w376 w380 w384]
                  tunnel: w354 -> [_ w363 w367 w371 w375 w379 w383]
                  frame 0, Default {
                    n254 = One Button Dialog(message="Choose filter first!") -> ()  [unwired: 2 out]
                  }
                  frame 1 {
                    n255 = Build Array(w365, w364, w363) -> (w362:dbl[])
                    n256 = local write "FLExposureTime"(w362) -> ()
                    n257 = global write "ProSCI Global.vi" "gFLExpTime"(w362) -> ()
                  }
                  frame 2 {
                    n258 = Build Array(w369, w368, w367) -> (w366:dbl[])
                    n259 = local write "FLExposureTime"(w366) -> ()
                    n260 = global write "ProSCI Global.vi" "gFLExpTime 2"(w366) -> ()
                  }
                  frame 3 {
                    n261 = Build Array(w373, w372, w371) -> (w370:dbl[])
                    n262 = local write "FLExposureTime"(w370) -> ()
                    n263 = global write "ProSCI Global.vi" "gFLExpTime 3"(w370) -> ()
                  }
                  frame 4 {
                    n264 = Build Array(w377, w376, w375) -> (w374:dbl[])
                    n265 = local write "FLExposureTime"(w374) -> ()
                    n266 = global write "ProSCI Global.vi" "gFLExpTime 4"(w374) -> ()
                  }
                  frame 5 {
                    n267 = Build Array(w381, w380, w379) -> (w378:dbl[])
                    n268 = local write "FLExposureTime"(w378) -> ()
                    n269 = global write "ProSCI Global.vi" "gFLExpTime 5"(w378) -> ()
                  }
                  frame 6 {
                    n270 = Build Array(w385, w384, w383) -> (w382:dbl[])
                    n271 = local write "FLExposureTime"(w382) -> ()
                    n272 = global write "ProSCI Global.vi" "gFLExpTime 6"(w382) -> ()
                  }
                }
              }
              frame #3 {
                n273 = global write "ProSCI Global.vi" "gFlExpMem"(w387) -> ()
                n274 = Wait (ms)(milliseconds to wait=u32 50) -> ()  [unwired: 1 out]
              }
            }
          }
          frame #1 {
            n275 = call "subVI QCam Get Exposures.vi"("error In"=w392, "cameraId In"=w393) -> ("qExposure Blue"=w388:dbl, "qExposure Red"=w389:dbl, "qExposure"=w390:dbl)  [unwired: 2 out]
            n276 = Build Array(w390, w389, w388) -> (w391:dbl[])
            n277 = local write "FL Exp"(w390) -> ()
            n278 = global write "ProSCI Global.vi" "gCurrentExpTime"(w391) -> ()
            n279 = local write "FL Blue Exp"(w388) -> ()
            n280 = local write "FL Red Exp"(w389) -> ()
          }
          frame #2 {
            n281 = local write "Stream"(TRUE ("Stream")) -> ()
          }
        }
      }
      event "SetBFExpsureTime": Value Change {
        n282 = event-data() -> ()  [unwired: 7 out]
        n283 = stacked-sequence {
          tunnel: w396 -> [w401 w431 _]
          tunnel: w395 -> [w400 w430 _]
          frame #0 {
            n284 = flat-sequence {
              tunnel: [w407] -> w399
              tunnel: [w406] -> w398
              tunnel: [w405] -> w397
              tunnel: [w419] -> w402
              tunnel: w401 -> [w421]
              tunnel: w400 -> [w420]
              tunnel: w399 -> [w419]
              tunnel: w398 -> [w418]
              tunnel: w397 -> [w417]
              tunnel: w402 -> [w425]
              frame #0 {
                n285 = local write "Stream"(FALSE ("Stream")) -> ()
              }
              frame #1 {
                n286 = local read "User Exp"() -> (w404:dbl)
                n287 = case shown="True" "Link Exposures (BF)" {
                  tunnel: [w409 w414] -> w407
                  tunnel: [w411 w416] -> w406
                  tunnel: [w410 w415] -> w405
                  tunnel: w404 -> [w409 w414]
                  frame False {
                    n288 = local read "User Blue Exp"() -> (w410:dbl)
                    n289 = local read "User Red Exp"() -> (w411:dbl)
                  }
                  frame True {
                    n290 = local read "Ratio BlueGreen"() -> (w412:dbl)
                    n291 = local read "Ratio RedGreen"() -> (w413:dbl)
                    n292 = Multiply(x=w413, y=w414) -> (x*y=w416:dbl)
                    n293 = Multiply(x=w412, y=w414) -> (x*y=w415:dbl)
                  }
                }
              }
              frame #2 {
                n294 = call "subVI QCam Set Exposures.vi"("qExposure"=w419, "qExposure Red"=w418, "cameraId In"=w421, "error In"=w420, "qExposure Blue"=w417, "Set Which Exposure"=enum16{"All", "Green", "Red", "Blue"}."All") -> ()  [unwired: 2 out]
                n295 = Build Array(w419, w418, w417) -> (w423:dbl[])
                n296 = global write "ProSCI Global.vi" "gBFExpTime"(w423) -> ()
              }
              frame #3 {
                n297 = global write "ProSCI Global.vi" "gBrExpMem"(w425) -> ()
                n298 = Wait (ms)(milliseconds to wait=u32 50) -> ()  [unwired: 1 out]
              }
            }
          }
          frame #1 {
            n299 = call "subVI QCam Get Exposures.vi"("error In"=w430, "cameraId In"=w431) -> ("qExposure Blue"=w426:dbl, "qExposure Red"=w427:dbl, "qExposure"=w428:dbl)  [unwired: 2 out]
            n300 = Build Array(w428, w427, w426) -> (w429:dbl[])
            n301 = global write "ProSCI Global.vi" "gCurrentExpTime"(w429) -> ()
            n302 = disable-structure shown="Disabled" {
              disable-tunnel: w428 -> [w434 _]
              disable-tunnel: w427 -> [w433 _]
              disable-tunnel: w426 -> [w432 _]
              frame Disabled {
                n303 = local write "User Exp"(w434) -> ()
                n304 = local write "User Red Exp"(w433) -> ()
                n305 = local write "User Blue Exp"(w432) -> ()
              }
              frame Enabled {
              }
            }
          }
          frame #2 {
            n306 = local write "Stream"(TRUE ("Stream")) -> ()
          }
        }
      }
      event "ForwardDelay": Value Change {
        n307 = event-data() -> ()  [unwired: 7 out]
        n308 = global write "ProSCI Global.vi" "gForwardDelay"("ForwardDelay") -> ()
      }
      event "PreImagingDelay": Value Change {
        n309 = event-data() -> ()  [unwired: 7 out]
        n310 = global write "ProSCI Global.vi" "gPreImagingDelay"("PreImagingDelay") -> ()
      }
      event "BFLampOnDelay": Value Change {
        n311 = event-data() -> ()  [unwired: 7 out]
        n312 = global write "ProSCI Global.vi" "gBFLampOnDelay"("BFLampOnDelay") -> ()
      }
      event "BFLampOffDelay": Value Change {
        n313 = event-data() -> ()  [unwired: 7 out]
        n314 = global write "ProSCI Global.vi" "gBFLampOffDelay"("BFLampOffDelay") -> ()
      }
      event "FLLampOnDelay": Value Change {
        n315 = event-data() -> ()  [unwired: 7 out]
        n316 = global write "ProSCI Global.vi" "gFLLampOnDelay"("FLLampOnDelay") -> ()
      }
      event "FLLampOffDelay": Value Change {
        n317 = event-data() -> ()  [unwired: 7 out]
        n318 = global write "ProSCI Global.vi" "gFLLampOffDelay"("FLLampOffDelay") -> ()
      }
    }
  }
  n319 = while {
    tunnel: w6 -> [w452]
    tunnel: w17 -> [w450]
    shift-right: [w448] -> _
    shift-left: _ -> [w449]
    tunnel: [w445] -> w19
    tunnel: [w444] -> w18
    tunnel: [w442] -> w9
    stop <- w442 stop-if-true
    # "If Image Type\nchanges between\nColor/Mono"
    n320 = local read "TypeChanged"() -> (w453:bool)
    n321 = local read "ColorImage"() -> (w451:T3)
    n322 = Wait (ms)(milliseconds to wait=u32 10) -> ()  [unwired: 1 out]
    n323 = case shown="False" w453 {
      tunnel: w452 -> [w589 w605]
      tunnel: w451 -> [w590 w604]
      tunnel: [w588 w603] -> w446
      tunnel: [w587 w602] -> w447
      tunnel: [w591 w601] -> w448
      tunnel: w450 -> [w586 _]
      tunnel: w449 -> [w585 _]
      frame False {
        n324 = local read "FirstPass"() -> (w592:bool)
        n325 = case shown="True" w592 {
          tunnel: [w595 w599] -> w591
          tunnel: w590 -> [_ w599]
          tunnel: w589 -> [w593 w600]
          tunnel: [w593 w598] -> w588
          tunnel: [w594 w597] -> w587
          tunnel: w586 -> [w594 w596]
          tunnel: w585 -> [w595 _]
          frame False {
            # "Do nothing, work with the last image type"
          }
          frame True {
            # "In first pass set up for Color"
            n326 = call "subVI QCam Change Image Type.vi"("error in"=w596, "Image In"=w599, "cameraId In"=w600) -> ("error out"=w597:errorcluster, "cameraId out"=w598:u32)
          }
        }
      }
      frame True {
        n327 = stacked-sequence {
          tunnel: w605 -> [w612 _]
          tunnel: w604 -> [w611 _]
          tunnel: [w610 _] -> w603
          tunnel: [w609 _] -> w602
          tunnel: [w608 _] -> w601
          frame #0 {
            # "Setup Grab for Color or Mono, depending on what has been chosen"
            n328 = Not Equal To 0?(x="qImage Type") -> (x != 0?=w606:bool)
            n329 = global write "ProSCI Global.vi" "gImageMono"(w606) -> ()
            n330 = case shown="\"Color\", Default" "qImage Type" {
              tunnel: [w613 w614] -> w608
              tunnel: w611 -> [w613 _]
              frame "Color", Default {
              }
              frame "Grayscale" {
                n331 = local read "MonoImage"() -> (w614:T3)
              }
            }
            n332 = call "subVI QCam Change Image Type.vi"("Image In"=w608, "cameraId In"=w612) -> ("error out"=w609:errorcluster, "cameraId out"=w610:u32)  [unwired: 1 in]
          }
          frame #1 {
            n333 = local write "TypeChanged"(FALSE) -> ()
          }
        }
      }
    }
    n334 = stacked-sequence {
      seq-local: [w457 _ _ _ _] -> [_ w473 _ _ _]
      seq-local: [w456 _ _ _ _] -> [_ w472 _ _ _]
      seq-local: [w455 _ _ _ _] -> [_ w471 _ _ _]
      seq-local: [_ w473 _ _ _] -> [_ _ w475 _ _]
      seq-local: [_ w472 _ _ _] -> [_ _ w490 _ _]
      seq-local: [_ w471 _ _ _] -> [_ _ w489 _ _]
      seq-local: [_ _ w474 _ _] -> [_ _ _ w501 _]
      seq-local: [_ _ w490 _ _] -> [_ _ _ w500 _]
      seq-local: [_ _ w489 _ _] -> [_ _ _ w495 _]
      tunnel: w448 -> [w460 _ _ _ _]
      tunnel: w447 -> [w459 _ w476 _ _]
      tunnel: w446 -> [w458 _ _ _ _]
      tunnel: [_ _ _ w495 _] -> w445
      tunnel: [_ _ _ w499 _] -> w444
      tunnel: [_ _ _ _ w583] -> w442
      frame #0 {
        n335 = local read "Stream"() -> (w454:bool)
        n336 = case shown="True" w454 {
          tunnel: w460 -> [w462 w469]
          tunnel: w459 -> [w461 w468]
          tunnel: w458 -> [w463 w467]
          tunnel: [w462 w466] -> w457
          tunnel: [w461 w465] -> w456
          tunnel: [w463 w464] -> w455
          frame False {
          }
          frame True {
            n337 = call "subVI QCam Grab Frame.vi"("error in"=w468, "Image Pointer In"=w469, "cameraId"=w467) -> ("error out"=w465:errorcluster, "Image Pointer Out"=w466:T3, "cameraId out"=w464:u32)
          }
        }
      }
      frame #1 {
        n338 = global write "ProSCI DebugGlobal.vi" "gDebug"("QCamera Frame 1" ("gDebug")) -> ()
      }
      frame #2 {
        # "This was for debugging"
        n339 = global write "QCam Color Globals.vi" "Green SW Gain"("Green Gain") -> ()
        n340 = global write "QCam Color Globals.vi" "Blue SW Gain"("Blue Gain") -> ()
        n341 = global write "QCam Color Globals.vi" "Red SW Gain"("Red Gain") -> ()
        n342 = Bundle By Name(cluster=T8 {"Green Exposure"=0.0, "Red Exposure"=0.0, "Blue Exposure"=0.0} ("Exposures"), "Green Exposure"="Green Exposure", "Red Exposure"="Red Exposure", "Blue Exposure"="Blue Exposure") -> (w483:T8)
        n343 = Bundle By Name(cluster=T7 {"Green Gain"=1, "Red Gain"=1, "Blue Gain"=1} ("Gains"), "Green Gain"="Green Gain", "Red Gain"="Red Gain", "Blue Gain"="Blue Gain") -> (w481:T7)
        n344 = call <userlib>:"QCAM Color Snap.vi"("New Image"=w475, "Exposures"=w483, "Gains"=w481, "error in (no error)"=w476) -> ("Image Out"=w474:T3, "error out"=w480:errorcluster)  [unwired: 5 in, 5 out]
        "Real-Time Image" <- w474
        n345 = flat-sequence {
          tunnel: w480 -> [w493]
          tunnel: [w493] -> _
          frame #0 {
            n346 = local read "Images Collected"() -> (w492:u64)
            n347 = Increment(x=w492) -> (x+1=w491:u64)
            n348 = local write "Images Collected"(w491) -> ()
          }
        }
        n349 = case shown="False" "Case Constant\n(See Context Help) 2" {
          frame False {
          }
          frame True {
            n350 = call "Subvi Event Log.vi"("EventNum"=u32 28) -> ()  [unwired: 1 in]
          }
        }
      }
      frame #3 {
        n351 = global read "ProSCI Global.vi" "gGrabImage"() -> (w503:bool)
        n352 = And(x=FALSE, y="Snap") -> (x .and. y?=w496:bool)
        n353 = Or(x=w503, y=w496) -> (x .or. y?=w502:bool)
        n354 = case shown="False" w502 {
          tunnel: w501 -> [w506 w511]
          tunnel: w500 -> [w504 w510]
          tunnel: [w504 w509] -> w499
          tunnel: w495 -> [_ w508]
          frame False {
            n355 = String To Path(string="\\\\csehomes\\csehome$\\dsp15\\Desktop\\testYDC.tif") -> (path=w507:path)
            n356 = call "IMAQ Write TIFF File"("File Path"=w507, "Image"=w506) -> ()  [unwired: 3 in, 4 out]
          }
          frame True {
            n357 = stacked-sequence {
              tunnel: [w515 _ _ _ _] -> w509
              tunnel: w511 -> [w513 w520 _ _ w565]
              tunnel: w510 -> [w512 _ _ _ _]
              tunnel: w508 -> [_ _ _ w563 _]
              frame #0 {
                n358 = global read "ProSCI Global.vi" "gFullFileName"() -> (w514:string)
                n359 = String To Path(string=w514) -> (path=w516:path)
                n360 = call "IMAQ Write TIFF File"("error in (no error)"=w512, "File Path"=w516, "Image"=w513) -> ("error out"=w515:errorcluster)  [unwired: 2 in, 3 out]
                "last image" <- w515
                n361 = case shown="Error" w515 {
                  frame No Error {
                    n362 = global write "ProSCI Global.vi" "gImageTaken"(TRUE) -> ()
                  }
                  frame Error {
                    n363 = global write "ProSCI Global.vi" "gImageTaken"(TRUE) -> ()
                    n364 = call "Subvi Event Log.vi"("EventNum"=u32 29) -> ()  [unwired: 1 in]
                  }
                }
              }
              frame #1 {
                n365 = local read "qImage Type"() -> (w521:enum32{"Color", "Grayscale"})
                n366 = case shown="\"Color\", Default" w521 {
                  tunnel: w520 -> [w525 w536]
                  frame "Color", Default {
                    n367 = flat-sequence {
                      tunnel: w525 -> [w529]
                      tunnel: [w529] -> w524
                      tunnel: [w527] -> w523
                      tunnel: [w526] -> w522
                      tunnel: w524 -> [w532]
                      tunnel: w523 -> [w531]
                      tunnel: w522 -> [w530]
                      frame #0 {
                        n368 = local read "Last Last Color"() -> (w528:T3)
                        n369 = local read "Last ColorImage"() -> (w527:T3)
                        n370 = call "IMAQ Copy"("Image Dst"=w528, "Image Src"=w527) -> ("error out"=w526:errorcluster)  [unwired: 1 in, 4 out]
                      }
                      frame #1 {
                        n371 = call "IMAQ Copy"("error in (no error)"=w530, "Image Dst"=w531, "Image Src"=w532) -> ()  [unwired: 5 out]
                      }
                    }
                  }
                  frame "Grayscale" {
                    n372 = flat-sequence {
                      tunnel: w536 -> [w540]
                      tunnel: [w540] -> w535
                      tunnel: [w538] -> w534
                      tunnel: [w537] -> w533
                      tunnel: w535 -> [w543]
                      tunnel: w534 -> [w542]
                      tunnel: w533 -> [w541]
                      frame #0 {
                        n373 = local read "Last MonoImage"() -> (w538:T3)
                        n374 = local read "Last Last Mono"() -> (w539:T3)
                        n375 = call "IMAQ Copy"("Image Dst"=w539, "Image Src"=w538) -> ("error out"=w537:errorcluster)  [unwired: 1 in, 4 out]
                      }
                      frame #1 {
                        n376 = call "IMAQ Copy"("error in (no error)"=w541, "Image Dst"=w542, "Image Src"=w543) -> ()  [unwired: 5 out]
                      }
                    }
                  }
                }
              }
              frame #2 {
                n377 = local read "qImage Type"() -> (w545:enum32{"Color", "Grayscale"})
                n378 = case shown="\"Color\", Default" w545 {
                  tunnel: [w548 w552] -> w546
                  tunnel: "Last Or Last Last" -> [w547 w551]
                  frame "Color", Default {
                    n379 = case shown="\"Last Last\"" w547 {
                      tunnel: [w549 w550] -> w548
                      frame "Last", Default {
                        n380 = local read "Last ColorImage"() -> (w549:T3)
                      }
                      frame "Last Last" {
                        n381 = local read "Last Last Color"() -> (w550:T3)
                      }
                    }
                  }
                  frame "Grayscale" {
                    n382 = case shown="\"Last Last\"" w551 {
                      tunnel: [w553 w554] -> w552
                      frame "Last", Default {
                        n383 = local read "Last MonoImage"() -> (w553:T3)
                      }
                      frame "Last Last" {
                        n384 = local read "Last Last Mono"() -> (w554:T3)
                      }
                    }
                  }
                }
                "Last Image" <- w546
                n385 = local write "Last Display Type"(w545) -> ()
              }
              frame #3 {
                w564 = FALSE
                # "Add dialog box here to check Exposure time for each snapped image"
                n386 = call "subVI QCam Get Exposures.vi"("cameraId In"=w563) -> ("qExposure Blue"=w560:dbl, "qExposure Red"=w561:dbl, "qExposure"=w562:dbl)  [unwired: 1 in, 2 out]
                n387 = Number To Fractional String(number=w562) -> (F-format string=w557:string)  [unwired: 3 out]
                n388 = Number To Fractional String(number=w561) -> (F-format string=w556:string)  [unwired: 3 out]
                n389 = Number To Fractional String(number=w560) -> (F-format string=w555:string)  [unwired: 3 out]
                n390 = global write "ProSCI Global.vi" "gGrabImage"(w564) -> ()
                n391 = local write "Snap"(w564) -> ()
                n392 = Concatenate Strings(w557, "/", w556, "/", w555) -> ()  [unwired: 1 out]
              }
              frame #4 {
                n393 = global read "ProSCI Global.vi" "gThumbThis"() -> (w566:bool)
                n394 = case shown="True" w566 {
                  tunnel: w565 -> [_ w567]
                  frame False {
                  }
                  frame True {
                    n395 = stacked-sequence {
                      seq-local: [w571 _] -> [_ w581]
                      tunnel: w567 -> [w575 _]
                      frame #0 {
                        w578 = 8
                        n396 = call "IMAQ GetImageInfo"("Image"=w575) -> ("Y Resolution"=w576:i32, "X Resolution"=w577:i32, "Image Type"=w579:T5)  [unwired: 1 in, 7 out]
                        n397 = call "IMAQ Create"("Image Name"="Thumb", "Image Type"=w579) -> ("New Image"=w574:T3)  [unwired: 2 in, 2 out]
                        n398 = Divide(x=w577, y=w578) -> (x/y=w573:dbl)
                        n399 = Divide(x=w576, y=w578) -> (x/y=w572:dbl)
                        n400 = Temporary Directory() -> (w570:path)
                        n401 = Build Path(base path=w570, name or relative path="CryoThumb.jpg" ("Image Name")) -> (appended path=w568:path)
                        n402 = call "IMAQ Resample"("X Resolution"=w573, "Y Resolution"=w572, "Image Dst"=w574, "Image Src"=w575) -> ("Image Dst Out"=w571:T3)  [unwired: 3 in, 4 out]
                        n403 = call "IMAQ Write JPEG File"("File Path"=w568, "Image"=w571) -> ()  [unwired: 3 in, 4 out]
                      }
                      frame #1 {
                        n404 = global write "ProSCI Global.vi" "gThumbThis"(FALSE) -> ()
                        n405 = call "IMAQ Dispose"("Image"=w581) -> ()  [unwired: 2 in, 4 out]
                      }
                    }
                  }
                }
              }
            }
          }
        }
      }
      frame #4 {
        n406 = local write "FirstPass"(FALSE) -> ()
        n407 = local read "Stop Button"() -> (w583:bool)
      }
    }
  }
  n408 = while {
    shift-right: [w617] -> _
    shift-left: w7 -> [w619]
    stop <- w616 stop-if-true
    n409 = Wait (ms)(milliseconds to wait=u32 5) -> ()  [unwired: 1 out]
    n410 = global read "ProSCI Global.vi" "gFLExcitationFilter"() -> (w617:i8)
    n411 = Subtract(x=w617, y=w619) -> (x-y=w620:i32)
    n412 = Not Equal To 0?(x=w620) -> (x != 0?=w618:bool)
    n413 = case shown="False" w618 {
      tunnel: w617 -> [_ w623]
      frame False {
        n414 = global read "ProSCI Global.vi" "gCurrentExpTime"() -> (→"CurrentExposureTime":dbl[])
      }
      frame True {
        n415 = flat-sequence {
          tunnel: w623 -> [w625]
          frame #0 {
            w624 = FALSE
            n416 = local write "FLExciteLED3"(w624) -> ()
            n417 = local write "FLExciteLED1"(w624) -> ()
            n418 = local write "FLExciteLED2"(w624) -> ()
            n419 = local write "FLExciteLED4"(w624) -> ()
            n420 = local write "FLExciteLED5"(w624) -> ()
            n421 = local write "FLExciteLED6"(w624) -> ()
          }
          frame #1 {
            n422 = case shown="1, Default" w625 {
              frame 1, Default {
                "FLExciteLED1" <- TRUE
              }
              frame 2 {
                "FLExciteLED2" <- TRUE
              }
              frame 3 {
                "FLExciteLED3" <- TRUE
              }
              frame 4 {
                "FLExciteLED4" <- TRUE
              }
              frame 5 {
                "FLExciteLED5" <- TRUE
              }
              frame 6 {
                "FLExciteLED6" <- TRUE
              }
            }
          }
        }
      }
    }
    n423 = local read "Stop Button"() -> (w616:bool)
  }
  n424 = flat-sequence {
    tunnel: w19 -> [w634]
    tunnel: w18 -> [w633]
    tunnel: [w632] -> w2
    tunnel: w9 -> [w632]
    tunnel: w2 -> [w639]
    tunnel: [w639] -> w1
    tunnel: [w640] -> w10
    tunnel: w1 -> [w640]
    tunnel: w10 -> [w644]
    frame #0 {
      n425 = call "QCAM Grab Stop.vi"("error in (no error)"=w633, "cameraId"=w634) -> ("error out"=w637:errorcluster, "cameraId Out"=w638:u32)
      n426 = call "IMAQ Dispose"("All Images? (No)"=TRUE, "error in (no error)"=w637) -> ("error out"=w636:errorcluster)  [unwired: 1 in, 3 out]
      n427 = call "QCAM Close.vi"("error in (no error)"=w636, "cameraId"=w638) -> ()  [unwired: 1 out]
    }
    frame #1 {
      n428 = call "ExCloseGlobalCam.vi"() -> ()  [unwired: 1 in]
    }
    frame #2 {
      n429 = call "subVI QCam Save File Parameters.vi"("exposure Blue"="User Blue Exp", "exposure Red"="User Red Exp", "exposure"="User Exp") -> ()
    }
    frame #3 {
      n430 = stacked-sequence {
        tunnel: w644 -> [_]
        frame #0 {
          n431 = Current VI's Path() -> (path=w645:path)
          n432 = Open VI Reference(vi path=w645) -> (vi reference=w649:refnum<vi>, error out=w650:errorcluster)  [unwired: 1 in, 4 out]
          n433 = property class="VI"(reference=w649, error in=w650, "Front Panel Window:Open"=FALSE) -> (reference out=w647:refnum<vi>, error out=w648:errorcluster)
          n434 = Close Reference(reference=w647, error in (no error)=w648) -> ()  [unwired: 1 out]
        }
      }
    }
    frame #4 {
      n435 = global write "ProSCI Global.vi" "gAppsStopped"(u8 1 ("gAppsStopped")) -> ()
    }
  }
